vi "TDMS_open_and_plot.vi"() -> ()   [LabVIEW 2018]
uses:
  SubVi's/Controls/CTL_Loaded_data_output_(offline).ctl
  Tracker.lvlib
  <vilib>/Analysis/NI_AALBase.lvlib
  Common_Resources.lvlib
panel:
  out "Missing":i32
  out "Total":i32
  out "Out of band":u32[](array[numeric])
  out "Histogram Graph":T1(graph)
  out "Hw and SW timings plot":dbl[][](graph)
  out "group/channel names":string[][](array[string])
  out "group names":string[](array[string])
  out "Loaded data output":T2
  in  "File Path Control":path=path "D:/Users_Data/Dmitriy_T/Documents/F4/Work_Data/Dima Toptunov/Support/Dino Dvorak/mousey21/Max_Track_(ssd_new)_2019-11-14-11-59-06/track.tdms"
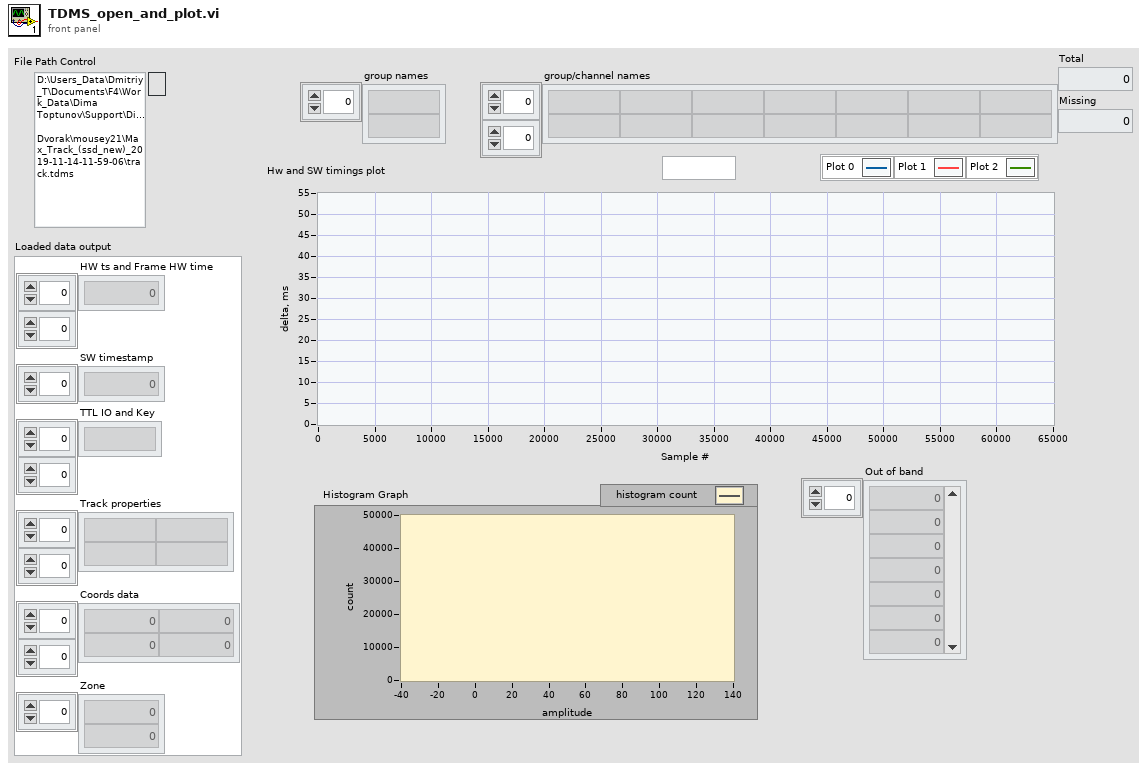
[diagram p1: front panel]
types:
  T1 = cluster{"X Values":dbl[], "Histogram: h(x)":i32[]}
  T2 = typedef "Common_Resources.lvlib/CTL_Loaded_data_output_(offline).ctl" = cluster{"HW ts and Frame HW time":u32[][], "SW timestamp":dbl[], "TTL IO and Key":string[][], "Track properties":string[][], "Coords data":dbl[][], "Zone":i8[]}
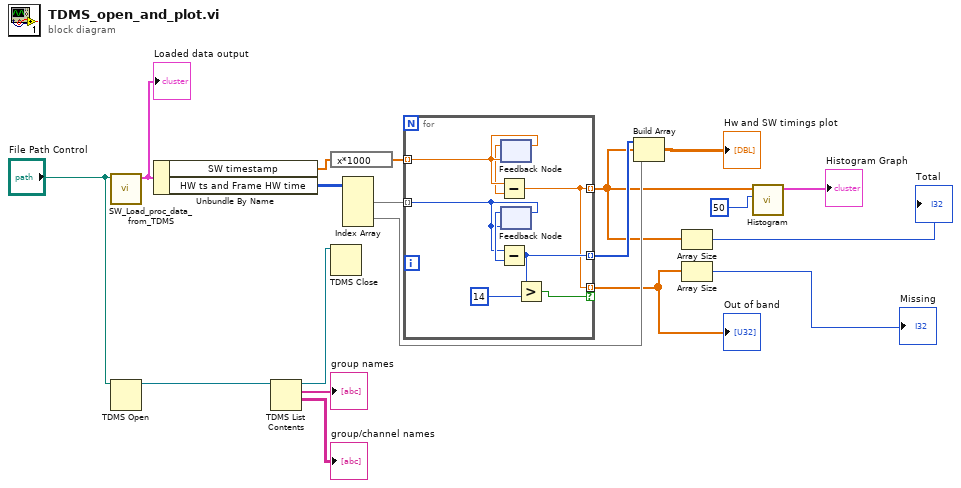
[diagram p0: block diagram]
diagram:
  n1 = call "SW_Load_proc_data_from_TDMS.vi"("TDMS track ref. in"="File Path Control") -> ("Loaded data output"=w15:T2)  [unwired: 8 in, 2 out]
  "Loaded data output" <- w15
  n2 = TDMS Open(11:"File Path Control") -> (3:w19:refnum<k34>)  [unwired: 6 in, 1 out]
  n3 = Unbundle By Name(w15) -> ("SW timestamp"=w13:dbl[], "HW ts and Frame HW time"=w9:u32[][])
  n4 = TDMS List Contents(7:w19) -> (1:→"group/channel names":string[][], 2:→"group names":string[], 3:w16:refnum<k34>)  [unwired: 2 in, 1 out]
  n5 = expression code="x*1000"(w13) -> (w10:dbl[])
  n6 = TDMS Close(11:w16) -> ()  [unwired: 1 in, 2 out]
  n7 = Index Array(array=w9) -> (element #1=w8:u32[], element #2=w5:u32[])  [unwired: 4 in]
  n8 = for {
    tunnel: w10 -> [w27] mode=indexing
    tunnel: [w20] -> w3 mode=indexing
    tunnel: w8 -> [w24] mode=indexing
    tunnel: [w23] -> w7 mode=indexing
    tunnel: [w20] -> w4 mode=indexing if=w21
    n9 = feedback-in #1(w27) -> ()
    n10 = feedback #1(w27) -> (w26:dbl)
    n11 = Subtract(x=w27, y=w26) -> (x-y=w20:dbl)
    n12 = feedback #2(w24) -> (w25:u32)
    n13 = Subtract(x=w24, y=w25) -> (x-y=w23:u32)
    n14 = feedback-in #2(w24) -> ()
    n15 = Greater?(x=w23, y=u32 14) -> (0:w21:bool)
  }
  "Out of band" <- w4
  n16 = Build Array(w7, w3, w5) -> (→"Hw and SW timings plot":dbl[][])
  n17 = Array Size(array=w3) -> (size(s)=→"Total":i32)
  n18 = Array Size(array=w4) -> (size(s)=→"Missing":i32)
  n19 = call <vilib>:"Histogram.vi"("intervals"=50, "X"=w3) -> ("Histogram Graph"=→"Histogram Graph":T1)  [unwired: 6 in, 3 out]
